vi "Read Power Supply Rejection Ratio Analysis.vi"(8 "error in (no error)":errorcluster, 11 "VISA resource name":refnum<visa-resource-name>) -> (0 "error out":errorcluster, 2 "Analysis Result":string[][](table), 3 "VISA resource name out":refnum<visa-resource-name>)   [LabVIEW 2017, in "Agilent 2000 3000 X-Series.lvlib"]
doc: "Returns data from the Power Supply Rejection Ratio (PSRR) power analysis. \n\nNote:\nThis VI is not supported by EDUX1052A/G, DSOX1202A/G, DSOX1204A/G models"
uses:
  Agilent 2000 3000 X-Series.lvlib
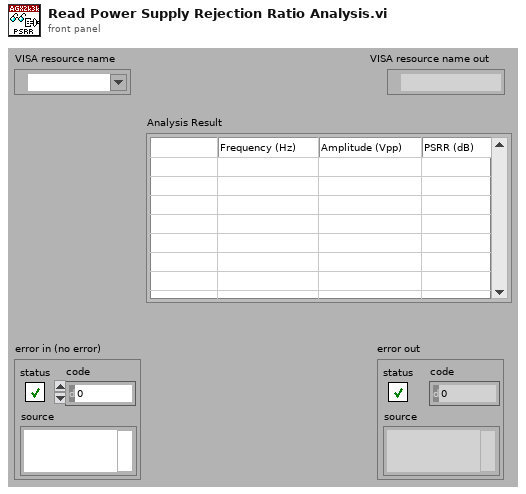
[diagram p1: front panel]
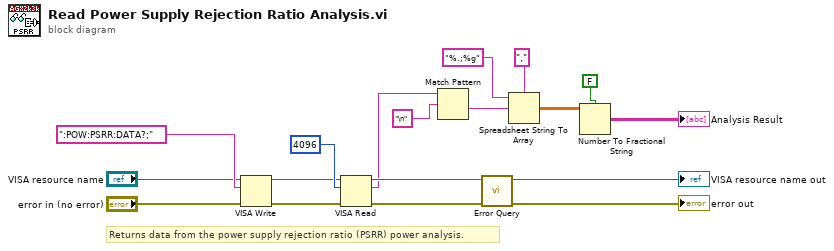
[diagram p0: block diagram]
diagram:
  # "Returns data from the power supply rejection ratio (PSRR) power analysis."
  n1 = VISA Write(VISA resource name="VISA resource name", write buffer=":POW:PSRR:DATA?;", error in (no error)="error in (no error)") -> (VISA resource name out=w14:refnum<visa-resource-name>, error out=w13:errorcluster)  [unwired: 1 out]
  n2 = VISA Read(VISA resource name=w14, byte count=4096, error in (no error)=w13) -> (VISA resource name out=w12:refnum<visa-resource-name>, read buffer=w3:string, error out=w11:errorcluster)  [unwired: 1 out]
  n3 = Match Pattern(string=w3, regular expression="\n") -> (after substring=w6:string)  [unwired: 1 in, 3 out]
  n4 = call "Error Query.vi"("error in (no error)"=w11, "VISA resource name"=w12) -> ("error out"=→"error out":errorcluster, "VISA resource name out"=→"VISA resource name out":refnum<visa-resource-name>)  [unwired: 6 in, 2 out]
  n5 = Spreadsheet String To Array(delimiter (Tab)=",", format string="%.;%g", spreadsheet string=w6) -> (array=w7:dbl[][])  [unwired: 1 in]
  n6 = Number To Fractional String(use system decimal point (T)=FALSE, number=w7) -> (F-format string=→"Analysis Result":string[][])  [unwired: 2 in]
